vi "Read DAQ DVR FIFO Direct Dispatch.vi"(8 "error in (no error)":errorcluster, 9 "Timeout (ms)":i32=100, 10 "Data In":refnum<data-value>[](array[refnum]), 11 "CIFTag in":refnum<class "CIFChannels.lvclass">) -> (0 "error out":errorcluster, 1 "timed out?":bool, 2 "Data Out":refnum<data-value>[](array[refnum]), 3 "CIFTag out":refnum<class "CIF_NIChn_Fifo_DAQ.lvclass">, 4 "Header":T1)   [LabVIEW 2021, in "CIF_NIChn_Fifo_DAQ.lvclass"]
uses:
  CIF_NIChn_Fifo_DAQ.lvclass
  D:/dev/CIF-LVCore/src/Channels/CIFChannels/CIFChannels.lvclass
  D:/dev/CIF-LVCore/src/Channels/CIF_NIChn/NIChn/CIF_NIChn.lvclass
  ChannelCommon/typedef/FIFO Header.ctl
  CIFChannels/CIFChannels.lvclass
  ChannelCommon/typedef/Datatype Waveform.ctl
  CIFChannels/CIFChannels.lvclass/CIFChannels.ctl
  NIChn/CIF_NIChn.lvclass/CIF_NIChn.ctl
  CIF_NIChn_Fifo_DAQ.lvclass/CIF_NIChn_Fifo_DAQ.ctl
  ChannelCommon/CIFFIFO/CIFfifo.lvclass/CIFfifo.ctl
  NIChn/Accessors/Read CIF Channel.vi
  NIChn/SubVIs/Check Disconnect.vi
  <vilib>/CIFChannels/Top Level/Read Variable Length U8 Array.vi
  NIChn/Accessors/Write CIF Channel.vi
  SubVIs/Unflatten.vi
  CIFChannels/Accessors/Read Channel State.vi
  CIFChannels/Accessors/Read Direction.vi
  CIFChannels/Accessors/Write Channel State.vi
  CIFChannels/Accessors/Read Disconnect Behavior.vi
  <vilib>/CIFChannels/Top Level/Read Variable Length U8 Array.vi/81056090-23cf-424a-a716-29db01c8ef1b.vi
  <vilib>/CIFChannels/Top Level/Read Variable Length U8 Array.vi/6610cd62-0a6d-4591-8fd4-6453482a4bc1.vi
  <vilib>/CIFChannels/Top Level/Read Variable Length U8 Array.vi/93d598b0-524b-4f76-9570-a74a86ef2c6f.vi
  ChannelCommon/CIFFIFO/Accessors/Write Timeout.vi
  ChannelCommon/CIFFIFO/Flatten/DVR Unflatten.vi
  ChannelCommon/CIFFIFO/Accessors/Read Header.vi
  ChannelCommon/CIFFIFO/Accessors/Write Header.vi
  <vilib>/CIFChannels/Top Level/Read Variable Length U8 Array.vi/81056090-23cf-424a-a716-29db01c8ef1b.vi/4bc1c15b-36ab-481f-b8dd-c64075ce723a.vi
  <vilib>/CIFChannels/Top Level/Read Variable Length U8 Array.vi/81056090-23cf-424a-a716-29db01c8ef1b.vi/d83cb72b-7713-41fc-a3d1-682de79cf574.vi
  <vilib>/CIFChannels/SubVIs/Get dll Path.vi
  <vilib>/CIFChannels/Top Level/Read Variable Length U8 Array.vi/6610cd62-0a6d-4591-8fd4-6453482a4bc1.vi/c28b0ead-42ad-4072-80a2-aca7f2bd7ce3.vi
  <vilib>/CIFChannels/Top Level/Read Variable Length U8 Array.vi/93d598b0-524b-4f76-9570-a74a86ef2c6f.vi/4bc1c15b-36ab-481f-b8dd-c64075ce723a.vi
  <vilib>/CIFChannels/Top Level/Read Variable Length U8 Array.vi/93d598b0-524b-4f76-9570-a74a86ef2c6f.vi/d83cb72b-7713-41fc-a3d1-682de79cf574.vi
  ChannelCommon/Utilities/Unflatten Header.vi
  CIFCore/Common/Utilities/Add Error.vi
  CIFCore/Common/Utilities/Append Error Location.vi
  NIChn/CIF_NIChn.lvclass
  ChannelCommon/ChannelCommon.lvlib
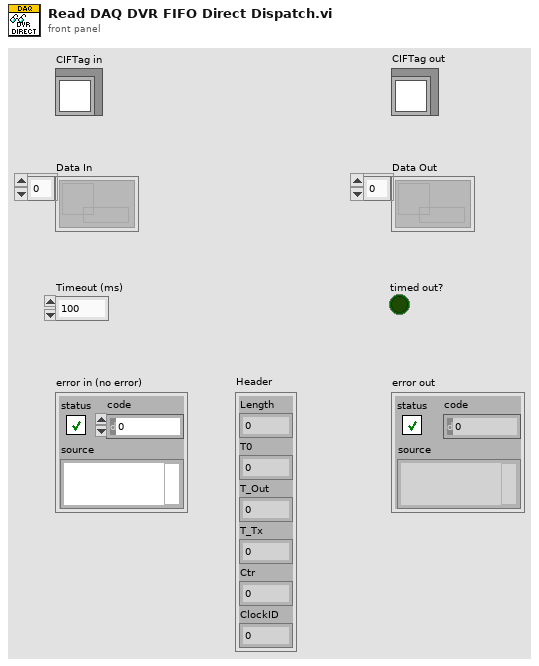
[diagram p1: front panel]
types:
  T1 = typedef "ChannelCommon.lvlib/FIFO Header.ctl" = cluster{"Length":u64, "T0":u64, "T_Out":u64, "T_Tx":u64, "Ctr":u64, "ClockID":u8}
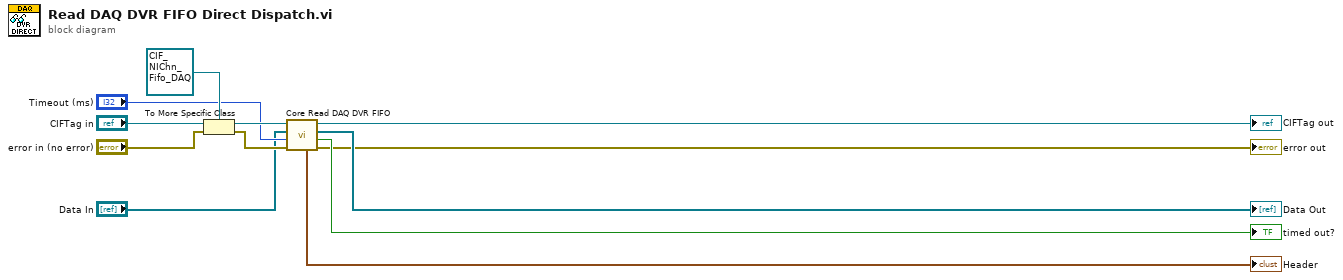
[diagram p0: block diagram]
diagram:
  n1 = To More Specific Class(target class=refnum<class "CIF_NIChn_Fifo_DAQ.lvclass"> refnum ("CIFTag in"), reference="CIFTag in", error in="error in (no error)") -> (specific class reference=w9:refnum<class "CIF_NIChn_Fifo_DAQ.lvclass">, error out=w7:errorcluster)
  n2 = call "Core Read DAQ DVR FIFO.vi"("error in (no error)"=w7, "Timeout (ms)"="Timeout (ms)", "Data In"="Data In", "CIFTag in"=w9) -> ("error out"=→"error out":errorcluster, "timed out?"=→"timed out?":bool, "Data Out"=→"Data Out":refnum<data-value>[], "CIFTag out"=→"CIFTag out":refnum<class "CIF_NIChn_Fifo_DAQ.lvclass">, "Header"=→"Header":T1)  [unwired: 3 in]
